vi "Terminate Data Queues.vi"(8 "error in (no error)":errorcluster, 11 "Task Base in":refnum<class "Task Base.lvclass">) -> (0 "error out":errorcluster, 3 "Task Base out":refnum<class "Task Base.lvclass">)   [LabVIEW 2023, in "HAL GOOP4.lvlib" / "Task Base.lvclass"]
uses:
  Task Base.lvclass
  Task Base.lvclass/Task Base.ctl
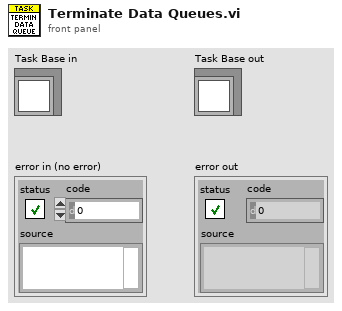
[diagram p1: front panel]
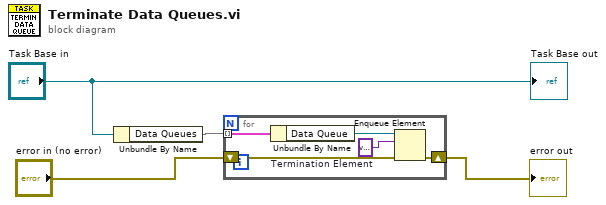
[diagram p0: block diagram]
diagram:
  n1 = Unbundle By Name("Task Base in") -> ("Data Queues"=w1:map{string, refnum<queue>})
  n2 = for {
    tunnel: w1 -> [w7] mode=indexing
    shift-right: [w8] -> w3
    shift-left: "error in (no error)" -> [w9]
    w6 = variant  # Termination Element
    n3 = Unbundle By Name(w7) -> ("Data Queue"=w5:refnum<queue>)
    n4 = Enqueue Element(queue=w5, element=w6, error in (no error)=w9) -> (error out=w8:errorcluster)  [unwired: 1 in, 2 out]
  }
  "error out" <- w3
  "Task Base out" <- "Task Base in"
